vi "MT Generate CPM Synchronization Parameters (number array).vi"(0 "CPM system parameters":T1={"samples per symbol (16)"=16, "symbol map"=[]}, 5 "sync numbers":i32[](array[numeric]) format="%.0x", 7 "bits per sync number":i32=32, 11 "error in (no error)":errorcluster, 12 "expected sync location (symbols)":i32=-1, 13 "sync location uncertainty (symbols)":i32=10, 14 "sync indent (symbols)":i32) -> (4 "CPM synchronization parameters":T2 {"sync sequence" format="%.2f"}, 15 "error out":errorcluster)   [LabVIEW 2020, in "niDMT.lvlib"]
doc: "This polymorphic instance generates synchronization parameters for CPM demodulation using a synchronization sequence defined by a <B>sync numbers</B> array in which each number represents a group of bits."
uses:
  <vilib>/addons/Modulation/niDMT.lvlib
  <vilib>/addons/Modulation/Digital/Support/Controls/CPM System Parameters.ctl
  <vilib>/addons/Modulation/niAMT.lvlib
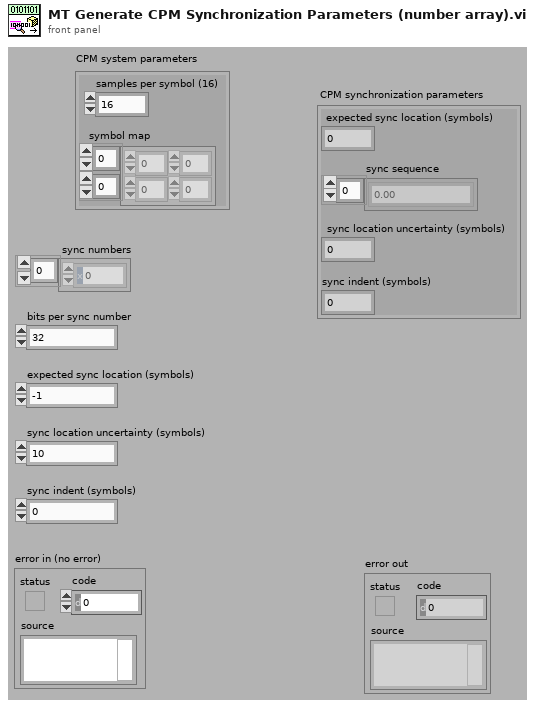
[diagram p1: front panel]
types:
  T1 = typedef "niDMT.lvlib/CPM System Parameters.ctl" = cluster{"samples per symbol (16)":i32, "symbol map":dbl[][]}
  T2 = cluster{"expected sync location (symbols)":i32, "sync sequence":cdb[], "sync location uncertainty (symbols)":i32, "sync indent (symbols)":i32}
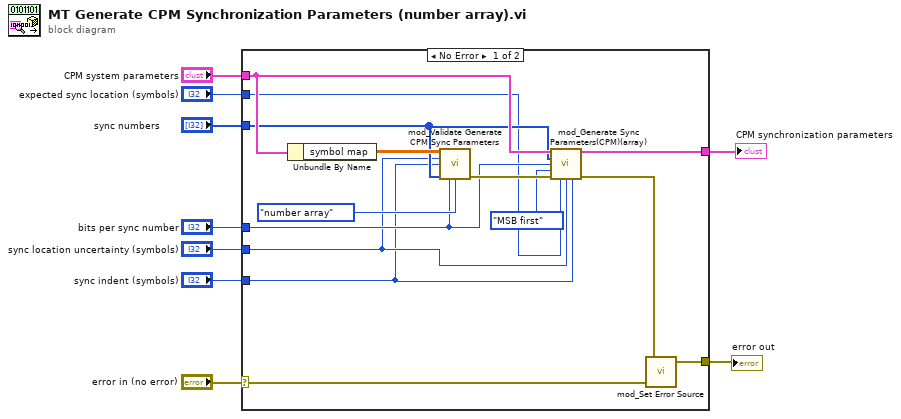
[diagram p0: block diagram]
diagram:
  n1 = case shown="No Error" "error in (no error)" {
    selector: "error in (no error)" -> [w22 w24]
    tunnel: "CPM system parameters" -> [w15 _]
    tunnel: "expected sync location (symbols)" -> [w10 _]
    tunnel: "sync location uncertainty (symbols)" -> [w12 _]
    tunnel: "sync indent (symbols)" -> [w11 _]
    tunnel: "sync numbers" -> [w14 _]
    tunnel: "bits per sync number" -> [w13 _]
    tunnel: [w23 w24] -> w2
    tunnel: [w19 _] -> w1
    frame No Error {
      n2 = Unbundle By Name(w15) -> ("symbol map"=w21:dbl[][])
      n3 = call <vilib>:"mod_Validate Generate CPM Sync Parameters.vi"("symbol map"=w21, "sync location uncertainty (symbols)"=w12, "sync indent (symbols)"=w11, "sync numbers"=w14, "number of bits (or) bits per number"=w13, "sync bits specification"=enum16{"bit array", "number array", "number"}."number array") -> ("error out"=w17:errorcluster)  [unwired: 1 in, 8 out]
      n4 = call <vilib>:"mod_Generate Sync Parameters(CPM)(array).vi"("CPM system parameters"=w15, "numbers"=w14, "bits per number"=w13, "bit order"=enum16{"MSB first", "LSB first"}."MSB first", "error in (no error)"=w17, "expected sync location (symbols)"=w10, "sync location uncertainty (symbols)"=w12, "sync indent (symbols)"=w11) -> ("CPM synchronization parameters"=w19:T2, "error out"=w18:errorcluster)  [unwired: 6 out]
      n5 = call <vilib>:"mod_Set Error Source.vi"("initial error in (no error)"=w22, "final error in (no error)"=w18) -> ("error out"=w23:errorcluster)  [unwired: 3 out]
    }
    frame Error {
    }
  }
  "CPM synchronization parameters" <- w1
  "error out" <- w2
